vi "Topo & GridSpectr_DriftCorrection_zSpec_v13.vi"(6 "Internal use":string, 7 "Grid param":T1 {"height (m)" format="%#_6p"; "width (m)" format="%#_6p"; "center Y (m)" format="%#_6p"; "center X (m)" format="%#_6p"}, 8 "Error in (no error)":errorcluster, 9 "Points Y/Index Y":i32, 10 "Points X/Index X":i32, 11 "Method":enum16{"init", "run", "end"}(ring)=enum."end") -> (0 "Error out":errorcluster)   [LabVIEW 2014]
doc: "Example of a measurement VI to be used in the \"Experiments on a Grid\" tool as external VI.\n\nThis example measure the topography and spectroscopy data. The spectroscopy measurements are taken on a subgrid. The data are saved to a sxm and a binary file.\n\n- Nanonis Programming Interface -"
uses:
  <userlib>/Nanonis Prog Interface V5/Scan/Grid/GridPatternGet.vi
  <userlib>/Nanonis Prog Interface V5/Scan/Grid/LinePatternGet.vi
  <userlib>/Nanonis Prog Interface V5/Nanonis Prog Interface.lvlib
panel:
  in  "during Spec Bias (V)":sgl=-0.00027 format="%#_5p"
  in  "type":u16(ring)=1 items=["Line", "Grid"]
  in  "readjust setpoint every":i32=4
  in  "Correct Drift":bool=TRUE
  in  "Email when finished":string="cornelius.krull@monash.edu"
  in  "STS z offset":dbl format="%#_6p"
  out "ETA":timestamp=timestamp(3568104746.9132867 s since 1904-01-01)
  out "remaining":dbl format="%<%H:%M:%S>t"
  out "Progress":u8(slide)=100 scale=0.0..100.0 scale format="%#.1g"
  out "total Points":i32=960
  in  "preSTS delay [ms]":u32=500
  in  "ref Bias":dbl=0.02 format="%#_6p"
  in  "Imaging Bias":dbl=0.02 format="%#_6p"
  in  "max applied Drift Correction":i32=20 min=1 max=100 step=1 format="%.0p"
  in  "Correlate":u16(ring) items=["first Frame", "successive Frames"]
  out "Topo Images taken":i32=47
  in  "Increment":i32=20
  in  "Threshold":i32=2 min=1 step=1
  in  "tip Speed (m/s)":sgl=2e-09 format="%.2p"
  out "X drift":i32=2
  out "Y drift":i32=-2
  out "Last Drift detected":i32=1
  in  "MaxImagesBack":i32=2
  in  "Channel index (0-23)":u8(ring) items=["Current"=0, "Z (m)"=14]
  in  "File name":string="symmetric_node"
  in  "ref Current":dbl=5e-12 format="%#_6p"
  in  "Imaging Current":dbl=5e-12 format="%#_6p"
  in  "zdrift \nDuration (s)":dbl
  in  "Correct z drift":bool
  out "Status":string="finishing"
  in  "Drift correction Pixels":i32=256 caption="Topo Pixels"
  out "Y Offset":dbl=3.096245239364581e-10 format="%#_6p"
  out "X Offset":dbl=3.3116363991336772e-09 format="%#_6p"
  out "Points taken":dbl=960.0
  in  "Drift Correction every":i32=20
  in  "Y subgrid spacing":u16=1
  in  "X subgrid spacing":u16=1
  # "z Spectroscopy"
  # "GRID points"
  # "Increase this if no Drift was detected for \na certain number of images"
  # "%"
  # "time (HH:MM:SS)"
  # "images back"
  # "% of image size"
  # "RUN smart tilt before starting the GRID\nImg Angle = 0\nmove tip to reference point for tip height"
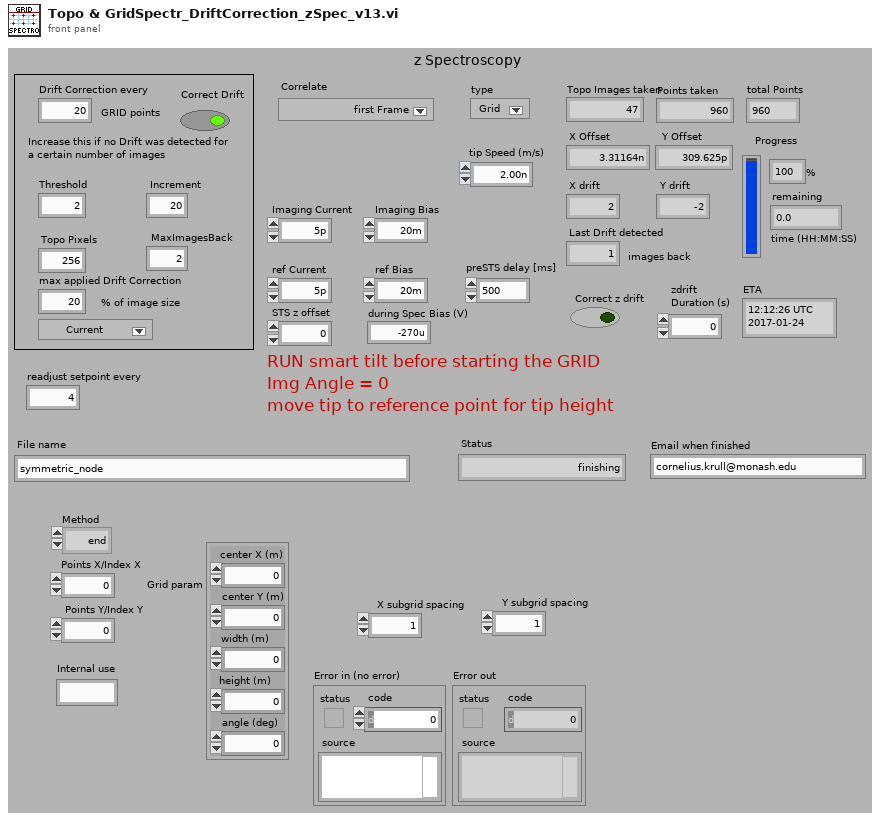
[diagram p1: front panel]
types:
  T1 = cluster{"center X (m)":sgl, "center Y (m)":sgl, "width (m)":sgl, "height (m)":sgl, "angle (deg)":sgl}
  T2 = cluster{"Z averaging time (s)":sgl, "Z offset (m)":sgl, "Initial settling time (s)":sgl}
  T3 = cluster{"Drift correction Pixels":i32, "Imaging Current":dbl, "STS Current":dbl, "MaxImagesBack":i32, "tip Speed (m/s)":sgl, "Threshold":i32, "Increment":i32, "Correlate":u16, "max applied Drift Correction":i32, "Imaging Bias":dbl, "Move Current":dbl, "Move Bias":dbl, "STS Bias":dbl, "preSTS delay [ms]":u32, "STS z offset":dbl, "Correct Drift":bool, "Lockin ON/OFF":bool}
  T4 = cluster{"center X":sgl, "center Y":sgl, "angle":sgl, "width":sgl, "height":sgl, "# pixels":i32, "# lines":i32}
  T5 = cluster{"Name":string, "Calibration":sgl, "Offset":sgl, "Channel index":i32}[]
  T6 = cluster{"up/down":bool, "time/line":sgl, "start time":timestamp, "end time":timestamp}
  T7 = cluster{"Z averaging time (s)":sgl, "Initial settling time (s)":sgl}
  T8 = cluster{"Max. slew rate (m/s)":sgl, "Settling time (s)":sgl, "Integration time (s)":sgl}
  T9 = cluster{"End settling time (s)":sgl, "Z control time (s)":sgl}
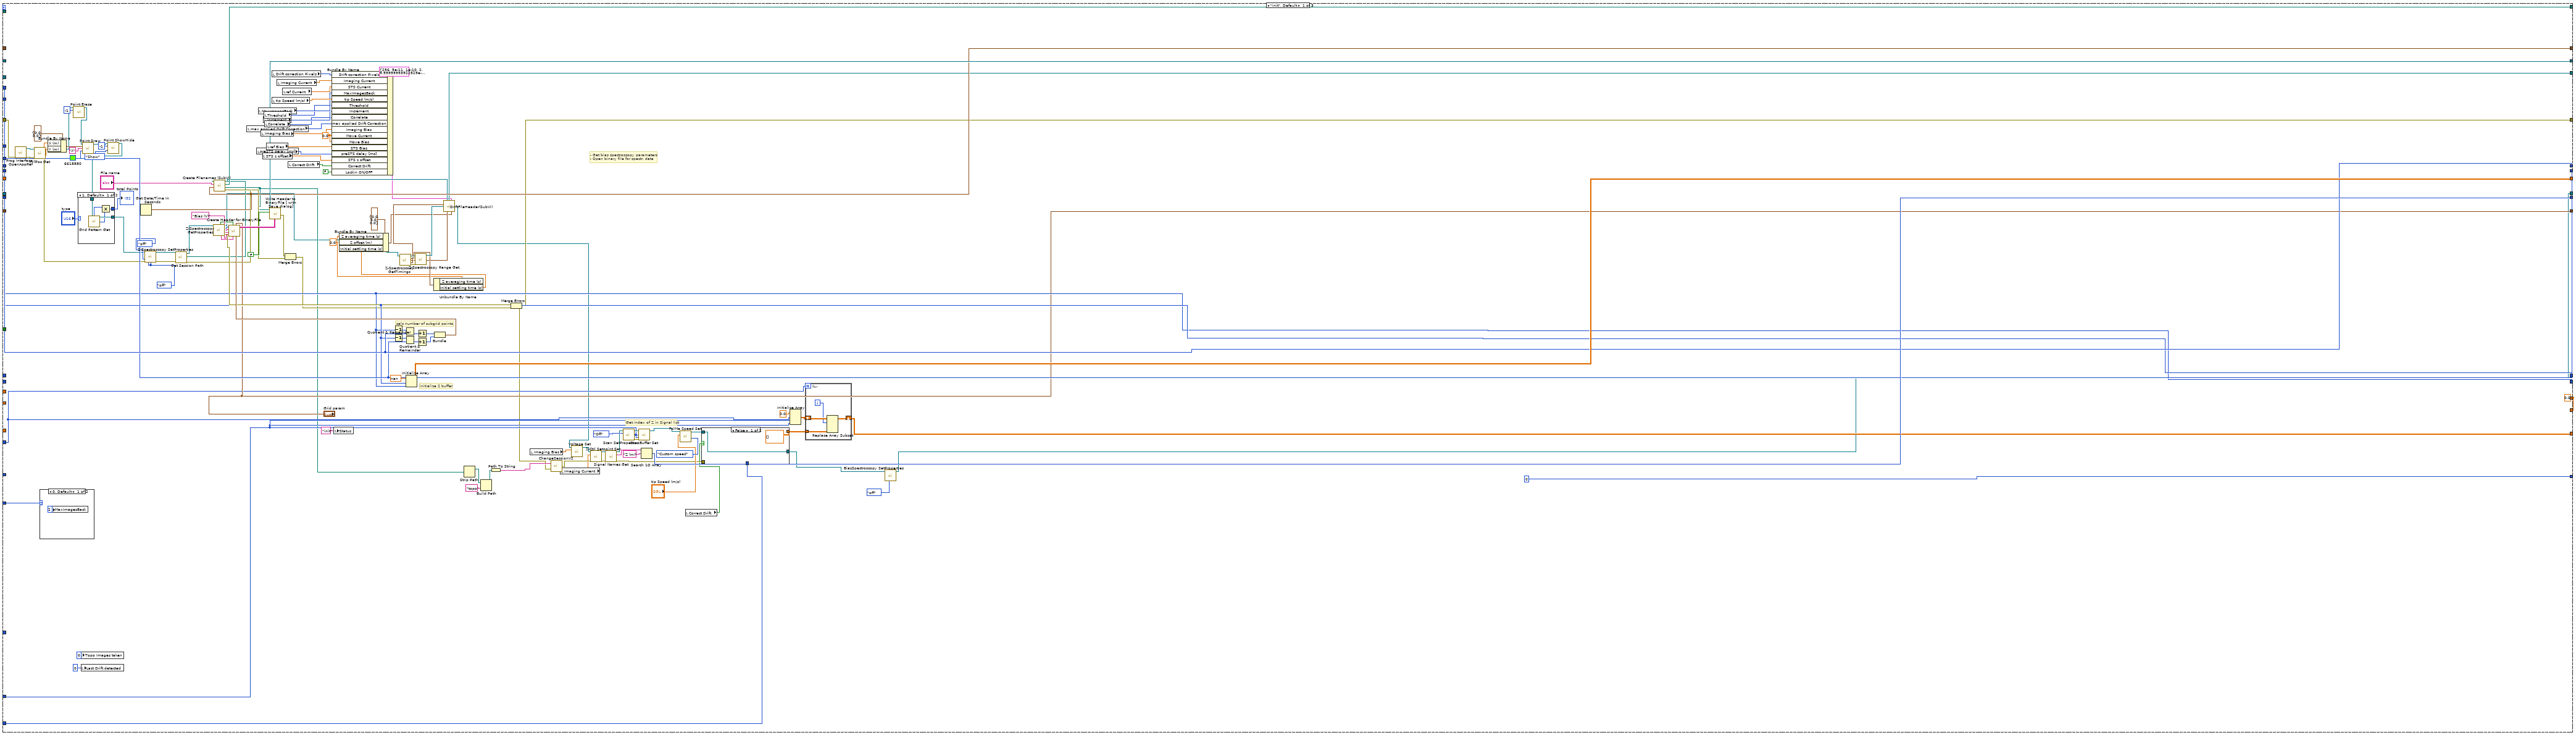
[diagram p2: hidden frame]
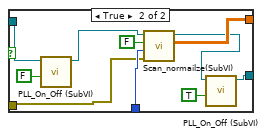
[diagram p3: hidden frame]
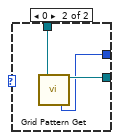
[diagram p4: hidden frame]
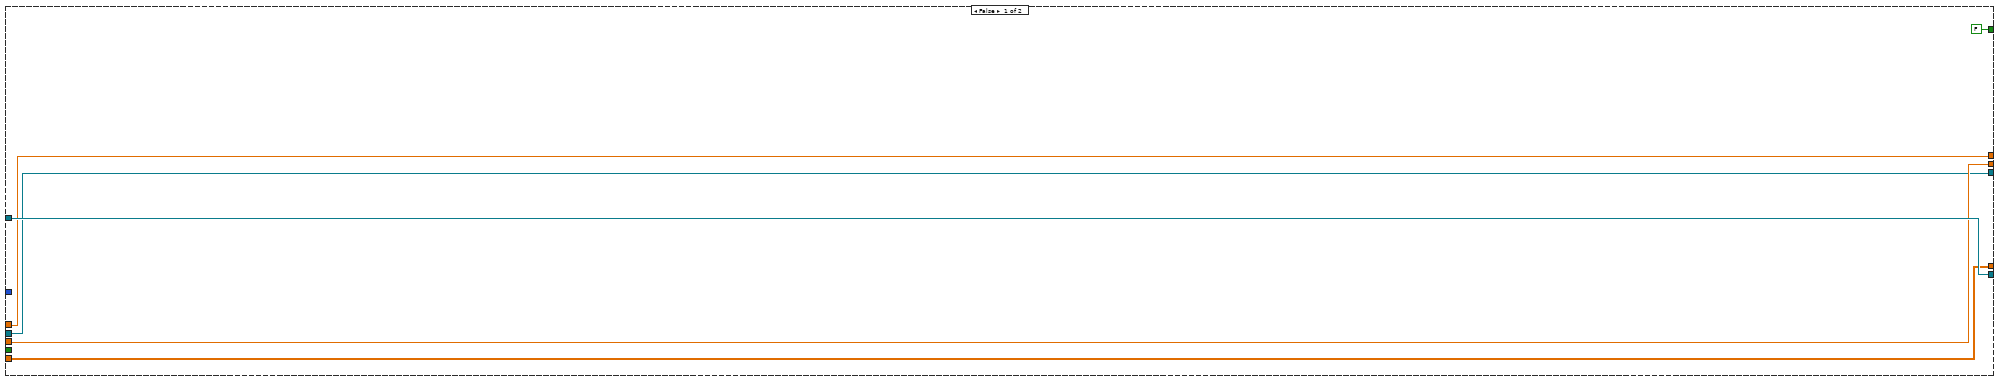
[diagram p9: hidden frame]
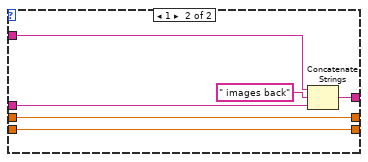
[diagram p10: hidden frame]
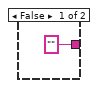
[diagram p12: hidden frame]
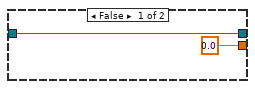
[diagram p13: hidden frame]
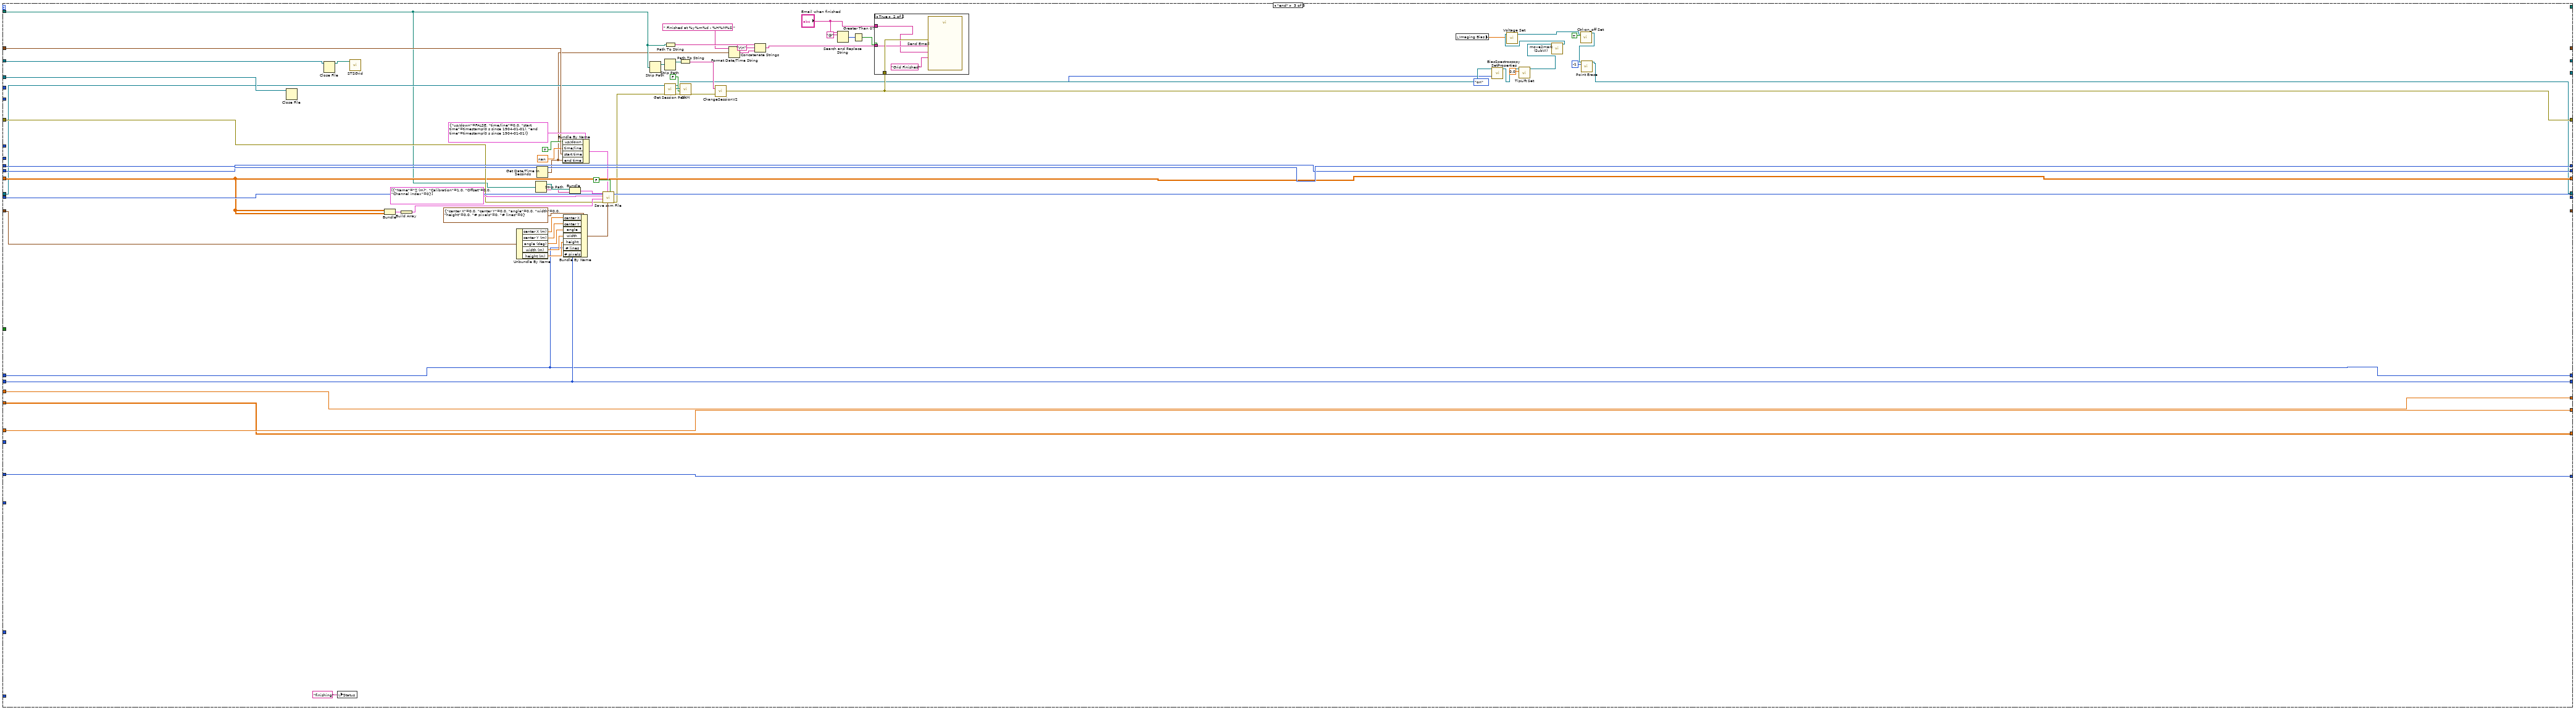
[diagram p15: hidden frame]
diagram:
  # "This string control is required so this VI's connector is compatible with the Nanonis module : \"Experiment on a grid\"."
  # "IMPORTANT : The connector of your own VI must EXACTLY match the connector of this example VI.\n\nThis example VI will do the following:\n- init: Open/Create a sxm (scan data file). Store file path in shift register. Initialize buffer for the topography data. Open binary file and create header.\n- run: Get Z position and write it to topography buffer (from last row to first row of buffer, to make it compatible to Save sxm File function which assumes data starting on the top left corner of image). If grid indices x,y are multiples of the subgrid spacings, start a bias spectroscopy experiment. Write the spectroscopy data to the binary file.\n- end: Write data from topography buffer to file, along with grid dimensions and other known parameters. Close files."
  n1 = while {
    shift-right: [w21] -> _
    shift-left: _ -> [w44]
    shift-right: [w39] -> _
    shift-left: _ -> [w38]
    shift-right: [w36] -> _
    shift-left: _ -> [w37]
    shift-right: [w35] -> _
    shift-left: _ -> [w34]
    shift-right: [w28] -> _
    shift-left: _ -> [w30]
    shift-right: [w29] -> _
    shift-left: _ -> [w31]
    shift-right: [w27] -> _
    shift-left: _ -> [w26]
    shift-right: [w25] -> _
    shift-left: _ -> [w24]
    shift-right: [w23] -> _
    shift-left: _ -> [w22]
    shift-right: [w20] -> _
    shift-left: _ -> [w19]
    shift-right: [w18] -> _
    shift-left: _ -> [w17]
    shift-right: [w16] -> _
    shift-left: _ -> [w9]
    shift-right: [w15] -> _
    shift-left: _ -> [w8]
    shift-right: [w14] -> _
    shift-left: _ -> [w11]
    shift-right: [w13] -> _
    shift-left: _ -> [w10]
    shift-right: [w6] -> _
    shift-left: _ -> [w5]
    stop <- TRUE stop-if-true
    # "> Drift file ref >"
    # "> number of  points  >"
    # "> Ref Frame  >"
    # "> Grid param >"
    # "> start time >"
    # ">Application reference >"
    # "> Y Subgrid spacing >"
    # "> X Subgrid spacing >"
    # "> Z signal index >"
    # "> Binary file ref >"
    # "> Z buffer >"
    # "> sxm file path >"
    n2 = case shown="\"run\"" "Method" {
      tunnel: [w139 w273 _] -> w21
      tunnel: w44 -> [_ w273 w449]
      tunnel: "Error in (no error)" -> [w141 w259 w480]
      tunnel: [w120 w272 w450] -> w42
      tunnel: "Points X/Index X" -> [w153 w267 _]
      tunnel: "Points Y/Index Y" -> [w154 w252 _]
      tunnel: [w177 w270 w469] -> w39
      tunnel: w38 -> [_ w271 w469]
      tunnel: w37 -> [_ w269 w462]
      tunnel: [w169 w268 _] -> w36
      tunnel: [w167 w257 w494] -> w35
      tunnel: w34 -> [_ w257 w494]
      tunnel: "X subgrid spacing" -> [w166 _ _]
      tunnel: "Y subgrid spacing" -> [w165 _ _]
      tunnel: w31 -> [_ w261 w493]
      tunnel: w30 -> [_ w260 w492]
      tunnel: [w166 w261 w493] -> w29
      tunnel: [w165 w260 w492] -> w28
      tunnel: [w105 w245 w433] -> w27
      tunnel: w26 -> [_ w229 w455]
      tunnel: ["Grid param" w255 _] -> w25
      tunnel: w24 -> [_ w255 w479]
      tunnel: [w138 w220 _] -> w23
      tunnel: w22 -> [_ w220 w487]
      tunnel: [w154 w253 w470] -> w20
      tunnel: w19 -> [_ w253 w470]
      tunnel: [w153 w254 w471] -> w18
      tunnel: w17 -> [_ w254 w471]
      tunnel: [w150 w235 w468] -> w16
      tunnel: [w150 w240 w466] -> w15
      tunnel: [w134 w234 w463] -> w14
      tunnel: [0 w218 w467] -> w13
      tunnel: w10 -> [_ w204 w467]
      tunnel: "Drift Correction every" -> [_ w248 _]
      tunnel: w11 -> [_ w239 w463]
      tunnel: w9 -> [_ w246 w468]
      tunnel: w8 -> [_ w232 w466]
      tunnel: "Drift correction Pixels" -> [w133 _ _]
      tunnel: [w101 w237 _] -> w6
      tunnel: w5 -> [_ w238 w464]
      tunnel: "Correct z drift" -> [_ w236 _]
      tunnel: "Channel index (0-23)" -> [w83 w233 _]
      tunnel: "MaxImagesBack" -> [w132 _ _]
      tunnel: "Correlate" -> [w113 _ _]
      frame "init", Default {
        w48 = 0.0 ("Move Current")
        w103 = enum16{"no change", "on", "off"}."off" ("Save dialog")
        w150 = 0.0
        # "- Get bias spectroscopy parameters\n- Open binary file for spectr. data"
        # "initialize Z buffer"
        # "calc number of subgrid points"
        # "Get index of Z in Signal list"
        n3 = call <userlib>:"Prog Interface - OpenAppRef.vi"("Error in (no error)"=w141) -> ("Error out"=w78:errorcluster, "Application reference"=w80:refnum<vi>)  [unwired: 5 in]
        n4 = call <userlib>:"XY-Pos Get.vi"("error in (no error)"=w78, "Application ref in"=w80) -> ("error out"=w79:errorcluster, "Y (m)"=w72:sgl, "X (m)"=w73:sgl, "Application ref out"=w54:refnum<vi>)  [unwired: 5 in]
        n5 = case shown="0, Default" w113 {
          frame 0, Default {
            n6 = local write "MaxImagesBack"(2 ("StepsBack")) -> ()
          }
          frame 1 {
          }
        }
        n7 = Bundle By Name(cluster=cluster{"X (m)":sgl, "Y (m)":sgl} {"X (m)"=0.0, "Y (m)"=0.0} ("Point Coordinates"), "X (m)"=w73, "Y (m)"=w72) -> (w74:cluster{"X (m)":sgl, "Y (m)":sgl})
        n8 = call <userlib>:"Point Erase.vi"("Application ref in"=w54, "Point index (-1=All points)"=-1) -> ("Application ref out"=w53:refnum<vi>)  [unwired: 12 in, 1 out]
        n9 = local write "Topo Images taken"(0 ("Images taken")) -> ()
        n10 = local write "Last Drift detected"(0 ("Last Drift detected")) -> ()
        n11 = call <userlib>:"Point Draw.vi"("Application ref in"=w53, "Point Coordinates"=w74, "Text"="X", "Color"=u32 6618880) -> ("Application ref out"=w58:refnum<vi>)  [unwired: 10 in, 1 out]
        n12 = call <userlib>:"Point ShowHide.vi"("Application ref in"=w58, "Point index (-1=All points)"=-1, "Show/Hide"=enum16{"Show", "Hide"}."Show") -> ("Application ref out"=w57:refnum<vi>)  [unwired: 11 in, 1 out]
        n13 = case shown="1, Default" "type" {
          tunnel: [w194 w197] -> w107
          tunnel: [w191 w195] -> w106
          tunnel: w57 -> [w190 w196]
          frame 1, Default {
            n14 = call-poly <userlib>:"Grid Pattern Get.vi"("Application ref in"=w190) -> ("Points Y"=w192:i32, "Points X"=w193:i32, "Application ref out"=w194:refnum<vi>)  [unwired: 10 in, 6 out]
            n15 = Multiply(x=w192, y=w193) -> (x*y=w191:i32)
          }
          frame 0 {
            n16 = call-poly <userlib>:"Grid Pattern Get.vi"("Application ref in"=w196) -> ("Points"=w195:i32, "Application ref out"=w197:refnum<vi>)  [unwired: 12 in, 5 out]
          }
        }
        "total Points" <- w106
        n17 = Get Date/Time In Seconds() -> (seconds since 1Jan1904=w138:timestamp)
        n18 = call <userlib>:"Z-Spectroscopy SetProperties.vi"("Application ref in"=w107, "Autosave"=enum16{"no change", "on", "off"}."off" ("Autosave (no change)"), "error in (no error)"=w79, "Save dialog"=w103, "Save all sweeps (no change)"=w103) -> ("Application ref out"=w116:refnum<vi>, "error out"=w115:errorcluster)  [unwired: 9 in]
        n19 = call <userlib>:"Get Session Path.vi"("error in (no error)"=w115, "Application ref in"=w116) -> ("error out"=w140:errorcluster, "Session path"=w126:path, "Application ref out"=w117:refnum<vi>)  [unwired: 7 in]
        n20 = call <userlib>:"Z-Spectroscopy GetProperties.vi"("Application ref in"=w117) -> ("Backward sweep"=w173:bool, "Application ref out"=w69:refnum<vi>, "Number of points"=w156:i32, "Channels"=w155:string[], "Parameters"=w171:string[], "Fixed parameters"=w158:string[], "error out"=w170:errorcluster)  [unwired: 7 in, 1 out]
        n21 = call "Create Filenames (SubVI).vi"("error in (no error)"=w140, "seconds since 1Jan1904"=w138, "File name"="File name", "Session path"=w126) -> ("error out"=w129:errorcluster, "binFilePath"=w122:path, "topoFilePath"=w139:path, "Drift File out"=w102:refnum<file>)  [unwired: 4 in]
        n22 = local read "max applied Drift Correction"() -> (w89:i32)
        n23 = local read "preSTS delay [ms]"() -> (w86:u32)
        n24 = local read "MaxImagesBack"() -> (w93:i32)
        n25 = local read "Imaging Bias"() -> (w88:dbl)
        n26 = local read "STS z offset"() -> (w85:dbl)
        n27 = local read "Increment"() -> (w91:i32)
        n28 = local read "Threshold"() -> (w92:i32)
        n29 = local read "Correlate"() -> (w90:u16)
        n30 = local read "ref Bias"() -> (w87:dbl)
        n31 = local read "Drift correction Pixels"() -> (w97:i32)
        n32 = local read "tip Speed (m/s)"() -> (w94:sgl)
        n33 = local read "Imaging Current"() -> (w96:dbl)
        n34 = local read "ref Current"() -> (w95:dbl)
        n35 = local read "Correct Drift"() -> (w84:bool)
        n36 = Bundle By Name(cluster=T3 {"Drift correction Pixels"=256, "Imaging Current"=5e-11, "STS Current"=1e-10, "MaxImagesBack"=2, "tip Speed (m/s)"=1e-08, "Threshold"=2, "Increment"=64, "Correlate"=0, "max applied Drift Correction"=20, "Imaging Bias"=-0.02, "Move Current"=1.5e-11, "Move Bias"=-0.02, "STS Bias"=0.1, "preSTS delay [ms]"=1000, "STS z offset"=-1.7e-10, "Correct Drift"=TRUE, "Lockin ON/OFF"=TRUE} ("Drift Correction"), "Drift correction Pixels"=w97, "Imaging Current"=w96, "STS Current"=w95, "MaxImagesBack"=w93, "tip Speed (m/s)"=w94, "Threshold"=w92, "Increment"=w91, "Correlate"=w90, "max applied Drift Correction"=w89, "Imaging Bias"=w88, "Move Current"=w48, "Move Bias"=w48, "STS Bias"=w87, "preSTS delay [ms]"=w86, "STS z offset"=w85, "Correct Drift"=w84, "Lockin ON/OFF"=FALSE) -> (w99:T3)
        n37 = local write "Status"("init" ("Status")) -> ()
        n38 = Decrement(x=w153) -> (x-1=w164:i32)
        n39 = Decrement(x=w154) -> (x-1=w163:i32)
        n40 = call <userlib>:"Z-Spectroscopy GetTimings.vi"("Application ref in"=w69) -> ("Application ref out"=w70:refnum<vi>, "Initialization"=w65:T7, "Sweep Timing"=w66:T8, "End of Sweep"=w67:T9, "Error out"=w71:errorcluster)  [unwired: 10 in]
        n41 = Quotient & Remainder(x=w164, y=w166) -> (floor(x/y)=w162:i32)  [unwired: 1 out]
        n42 = Quotient & Remainder(x=w163, y=w165) -> (floor(x/y)=w161:i32)  [unwired: 1 out]
        n43 = Initialize Array(sgl nan ("element"), w154, w153) -> (w177:sgl[][])
        n44 = call <userlib>:"Z-Spectroscopy Range Get.vi"("error in (no error)"=w71, "Application ref in"=w70) -> ("Application ref out"=w68:refnum<vi>)  [unwired: 5 in, 3 out]
        n45 = Increment(x=w162) -> (x+1=w160:i32)
        n46 = Increment(x=w161) -> (x+1=w159:i32)
        n47 = Unbundle By Name(w65) -> ("Z averaging time (s)"=w62:sgl, "Initial settling time (s)"=w61:sgl)
        n48 = Bundle By Name(cluster=T2 {"Z averaging time (s)"=0.0, "Z offset (m)"=0.0, "Initial settling time (s)"=0.0} ("Initialization"), "Z averaging time (s)"=w62, "Z offset (m)"=sgl 0.0, "Initial settling time (s)"=w61) -> (w63:T2)
        n49 = Bundle(w160, w159) -> (w172:cluster{i32, i32})  [unwired: 1 in]
        n50 = call <userlib>:"Create Header for BinaryFile.vi"("Grid points"=w172, "Grid param"="Grid param", "Fixed parameters"=w158, "Backward sweep"=w173, "Sweep signal"="Bias (V)" ("Sweep Signal"), "Parameters"=w171, "Channels"=w155, "Points per sweep"=w156) -> ("Header (fixed attributes)"=w175:string[][])  [unwired: 3 in]
        n51 = call <userlib>:"Write Header to BinaryFile [ with Save dialog].vi"("Fixed Attributes"=w175, "Show Dialog? (T)"=FALSE, "Filename"=w122) -> ("Error out"=w130:errorcluster, "File ref"=w169:refnum<file>)  [unwired: 5 in, 2 out]
        n52 = Merge Errors(w130, w129) -> (w131:errorcluster)
        n53 = call "DriftFileHeader(SubVI).vi"("Byte Stream File in"=w102, "Drift Correction"=w99, "End of Sweep"=w67, "Application ref in"=w68, "Sweep Timing"=w66, "Initialization"=w63) -> ("Byte Stream File out"=w101:refnum<file>, "Application ref out"=w100:refnum<vi>)  [unwired: 8 in]
        n54 = Strip Path(path=w122) -> (stripped path=w125:path)  [unwired: 1 out]
        n55 = Build Path(base path=w125, name or relative path="topo") -> (appended path=w123:path)
        n56 = Path To String(path=w123) -> (string=w121:string)
        n57 = Merge Errors(w170, w131) -> (w120:errorcluster)
        n58 = local read "Imaging Bias"() -> (w109:dbl)
        n59 = call "ChangeSessionV2.vi"("error in (no error)"=w120, "Session"=w121) -> ("error out"=w119:errorcluster)
        n60 = local read "Imaging Current"() -> (w108:dbl)
        n61 = call <userlib>:"Voltage Set.vi"("Bias (V)"=w109, "Application ref in"=w100) -> ("Application ref out"=w110:refnum<vi>)  [unwired: 8 in, 1 out]
        n62 = call <userlib>:"Z-Ctrl Setpoint Set.vi"("error in (no error)"=w119, "Z Controller setpoint"=w108, "Application ref in"=w110) -> ("error out"=w142:errorcluster, "Application ref out"=w143:refnum<vi>)  [unwired: 7 in]
        n63 = call <userlib>:"Signal Names Get.vi"("error in (no error)"=w142, "Application ref in"=w143) -> ("error out"=w82:errorcluster, "Signals Names"=w157:string[], "Application ref out"=w146:refnum<vi>)  [unwired: 5 in]
        n64 = call <userlib>:"Scan SetProperties.vi"("Application ref in"=w146, "Continuous scan"=enum16{"No change", "On", "Off"}."Off") -> ("Application ref out"=w148:refnum<vi>, "Error out"=w147:errorcluster)  [unwired: 12 in]
        n65 = call <userlib>:"ScanBuffer Set.vi"("Application ref in"=w148, "Pixels"=w133, "Lines"=w133, "error in (no error)"=w147) -> ("Application ref out"=w111:refnum<vi>)  [unwired: 10 in, 1 out]
        n66 = Search 1D Array(1D array=w157, element="Z (m)") -> (index of element=w167:i32)  [unwired: 1 in]
        n67 = call <userlib>:"FolMe Speed Set.vi"("Speed Setting (Custom)"=enum32{"Scan speed", "Custom speed"}."Custom speed", "Speed (m/s)"="tip Speed (m/s)", "Application ref in"=w111) -> ("Application ref out"=w51:refnum<vi>)  [unwired: 5 in, 1 out]
        n68 = local read "Correct Drift"() -> (w49:bool)
        n69 = case shown="False" w49 {
          tunnel: w83 -> [_ w189]
          tunnel: w82 -> [_ w188]
          tunnel: [dbl[][] [] ("Array") w187] -> w81
          tunnel: w51 -> [w179 w185]
          tunnel: [w179 w180] -> w47
          frame False {
          }
          frame True {
            n70 = call "PLL_On_Off (SubVI).vi"("Output ON/OFF (F=OFF)"=FALSE, "Application in"=w185) -> ("Application out"=w184:refnum<vi>)  [unwired: 8 in, 1 out]
            n71 = call "Scan_normailze(SubVI).vi"("error in (no error)"=w188, "Channel index (0-23)"=w189, "Normalization"=FALSE ("Boolean"), "Application in"=w184) -> ("Array"=w187:dbl[][], "Application out"=w181:refnum<vi>)  [unwired: 5 in, 1 out]
            n72 = call "PLL_On_Off (SubVI).vi"("Output ON/OFF (F=OFF)"=TRUE, "Application in"=w181) -> ("Application out"=w180:refnum<vi>)  [unwired: 8 in, 1 out]
          }
        }
        n73 = Initialize Array(0.0 ("element"), w132, w133, w133) -> (w135:dbl[][][])
        n74 = for {
          N: w132 -> [_]
          tunnel: w81 -> [w201]
          shift-right: [w200] -> w134
          shift-left: w135 -> [w202]
          i -> [w199]
          n75 = Replace Array Subset(array=w202, new element=w201, index (dim 0)=w199) -> (w200:dbl[][][])  [unwired: 2 in]
        }
        n76 = call <userlib>:"BiasSpectroscopy SetProperties.vi"("Application ref in"=w47, "Z-Controller hold (no change)"=enum16{"no change", "on", "off"}."off") -> ("Application ref out"=w105:refnum<vi>)  [unwired: 12 in, 1 out]
      }
      frame "run" {
        # "shift tip position"
        # "Get Z position"
        # "- get Z position for topography and store it to Z buffer\n- if x,y indices are a multiple of the spacings, take spectroscopy curve and write data to binary file\ndo drift correction if number of STS position was reached"
        n77 = local read "Correct Drift"() -> (w212:bool)
        n78 = Quotient & Remainder(x=w204, y=w248) -> (x-y*floor(x/y)=w249:i32)  [unwired: 1 out]
        n79 = Not Equal To 0?(x=w204) -> (x != 0?=w230:bool)
        n80 = Equal To 0?(x=w249) -> (x = 0?=w247:bool)
        n81 = call <userlib>:"XY-Pos Get.vi"("Wait for newest data (F=False)"=TRUE, "Application ref in"=w229) -> ("Y (m)"=w225:sgl, "X (m)"=w226:sgl, "Application ref out"=w228:refnum<vi>)  [unwired: 5 in, 1 out]
        n82 = Compound Arithmetic op=AND(w230, w247, w212) -> (w231:bool)
        n83 = case shown="True" w231 {
          tunnel: w228 -> [w314 w325]
          tunnel: [w314 w370] -> w209
          tunnel: w239 -> [w311 w366]
          tunnel: [w313 w368] -> w235
          tunnel: [w312 w367] -> w240
          tunnel: w246 -> [w313 w349]
          tunnel: w232 -> [w312 w347]
          tunnel: [w311 w362] -> w234
          tunnel: w238 -> [w310 w373]
          tunnel: [w310 w372] -> w237
          tunnel: w236 -> [_ w369]
          tunnel: w233 -> [_ w353]
          tunnel: [FALSE TRUE] -> w206
          frame False {
          }
          frame True {
            # "Drift correction \ncompare to the reference image with the previous image \ndx and dy will be applied to the grid coord, \nand the imaging frame will be shifted"
            n84 = Greater Or Equal To 0?(x=w353) -> (x >= 0?=w352:bool)
            n85 = call "move2mark (SubVI).vi"("Application in"=w325) -> ("Application out"=w324:refnum<vi>)  [unwired: 10 in]
            n86 = local write "Status"("Drift Correction" ("Status")) -> ()
            n87 = case shown="True" w352 {
              frame False {
              }
              frame True {
                n88 = local read "Topo Images taken"() -> (w388:i32)
                n89 = Increment(x=w388) -> (x+1=w387:i32)
                n90 = local write "Topo Images taken"(w387) -> ()
              }
            }
            n91 = local read "Imaging Bias"() -> (w332:dbl)
            n92 = call <userlib>:"Voltage Set.vi"("Bias (V)"=w332, "Application ref in"=w324) -> ("Application ref out"=w333:refnum<vi>)  [unwired: 8 in, 1 out]
            n93 = local read "Imaging Current"() -> (w331:dbl)
            n94 = call <userlib>:"Z-Ctrl Setpoint Set.vi"("Z Controller setpoint"=w331, "Application ref in"=w333) -> ("Application ref out"=w323:refnum<vi>)  [unwired: 8 in, 1 out]
            n95 = call <userlib>:"Ctrl-on_off Set.vi"("Z Controller ON/OFF"=TRUE, "Application ref in"=w323) -> ("Application ref out"=w321:refnum<vi>)  [unwired: 8 in, 1 out]
            n96 = call "PLL_On_Off (SubVI).vi"("Output ON/OFF (F=OFF)"=FALSE, "Application in"=w321) -> ("Application out"=w320:refnum<vi>)  [unwired: 8 in, 1 out]
            n97 = call "Scan_normailze(SubVI).vi"("Channel index (0-23)"=w353, "Normalization"=FALSE ("Boolean"), "Application in"=w320) -> ("Array"=w363:dbl[][], "Application out"=w318:refnum<vi>)  [unwired: 6 in, 1 out]
            n98 = Divide(x="max applied Drift Correction", y=100) -> (x/y=w340:dbl)
            n99 = local read "Drift correction Pixels"() -> (w341:i32)
            n100 = local read "Last Drift detected"() -> (w344:i32)
            n101 = local read "Correlate"() -> (w350:u16)
            n102 = call "PLL_On_Off (SubVI).vi"("Output ON/OFF (F=OFF)"=TRUE, "Application in"=w318) -> ("Application out"=w315:refnum<vi>)  [unwired: 8 in, 1 out]
            n103 = Multiply(x=w340, y=w341) -> (x*y=w342:dbl)
            n104 = call "CorrelImages (SubVI)v2.vi"("last drift detected"=w344, "Correlate"=w350, "Ref Array"=w366, "New Image"=w363) -> ("Y drift"=w338:i32, "X drift"=w335:i32, "Ref Array out"=w362:dbl[][][], "Queue Steps"=w351:i32)  [unwired: 4 in]
            "X drift" <- w335
            "Y drift" <- w338
            "Last Drift detected" <- w351
            n105 = local read "Topo Images taken"() -> (w355:i32)
            n106 = To Long Integer(number=w342) -> (32bit integer=w334:i32)
            n107 = Greater Or Equal?(x=w351, y="Threshold") -> (x >= y?=w357:bool)
            n108 = Greater?(x=w355, y="Threshold") -> (0:w354:bool)
            n109 = call "AbsLimit (SubVI).vi"("in"=w335, "Abslimt"=w334) -> ("Numeric out"=w337:i32)  [unwired: 9 in]
            n110 = call "AbsLimit (SubVI).vi"("in"=w338, "Abslimt"=w334) -> ("Numeric out"=w336:i32)  [unwired: 9 in]
            n111 = And(x=w357, y=w354) -> (x .and. y?=w356:bool)
            n112 = case shown="True" w356 {
              tunnel: ["" w392] -> w358
              frame False {
              }
              frame True {
                n113 = local read "Drift Correction every"() -> (w391:i32)
                n114 = local write "Last Drift detected"(0 ("Last Drift detected")) -> ()
                n115 = Add(x=w391, y="Increment") -> (x+y=w395:i32)
                n116 = local write "Drift Correction every"(w395) -> ()
                n117 = Number To Decimal String(number=w395) -> (decimal integer string=w394:string)  [unwired: 1 in]
                n118 = Concatenate Strings(" Increased DC to every " ("string"), w394) -> (w392:string)
              }
            }
            n119 = local read "Drift correction Pixels"() -> (w360:i32)
            n120 = Number To Decimal String(number=w351) -> (decimal integer string=w365:string)  [unwired: 1 in]
            n121 = case shown="0, Default" w350 {
              tunnel: w365 -> [w375 w386]
              tunnel: [w380 w385] -> w364
              tunnel: w358 -> [w378 w383]
              tunnel: w349 -> [w376 w382]
              tunnel: [w376 w382] -> w348
              tunnel: w347 -> [w377 w381]
              tunnel: [w377 w381] -> w346
              frame 0, Default {
                n122 = Concatenate Strings(w375, "images back , Correlating first frame " ("string"), w378) -> (w380:string)
              }
              frame 1 {
                n123 = Concatenate Strings(w386, " images back" ("string"), w383) -> (w385:string)
              }
            }
            n124 = call "drift_pixel2m (SubVI).vi"("Application in"=w315, "X drift"=w337, "Y drift"=w336, "Drift correction Pixels"=w360) -> ("Application out"=w359:refnum<vi>, "x drift"=w329:sgl, "y drift"=w328:sgl)  [unwired: 2 in, 1 out]
            n125 = call "ShiftFrame (SubVI).vi"("Y shift"=w328, "X shift"=w329, "Application in"=w359) -> ("Application out"=w361:refnum<vi>)  [unwired: 8 in]
            n126 = call "MoveGrid.vi"("y"=w328, "x"=w329, "Application ref in"=w361) -> ("Application ref out"=w327:refnum<vi>)  [unwired: 7 in, 1 out]
            n127 = call "shift marks (SubVI).vi"("y"=w328, "x"=w329, "Application in"=w327) -> ("Application out"=w326:refnum<vi>)  [unwired: 7 in, 1 out]
            n128 = case shown="True" w369 {
              tunnel: [0.0 ("z drift") w402] -> w371
              tunnel: w326 -> [w397 w401]
              tunnel: [w397 w400] -> w370
              frame False {
              }
              frame True {
                n129 = call "Zdrift_subVi.vi"("Duration"="zdrift \nDuration (s)", "Application in"=w401) -> ("z drift"=w402:dbl, "Application out"=w400:refnum<vi>)  [unwired: 7 in, 1 out]
              }
            }
            n130 = Add(x=w348, y=w329) -> (x+y=w368:dbl)
            n131 = Add(x=w328, y=w346) -> (x+y=w367:dbl)
            n132 = local write "X Offset"(w368) -> ()
            n133 = local write "Y Offset"(w367) -> ()
            n134 = call "Drift Data to file (SubVI).vi"("z drift"=w371, "Comment"=w364, "y Drift"=w367, "X drift"=w368, "Byte Stream File in"=w373) -> ("Byte Stream File out"=w372:refnum<file>)  [unwired: 6 in]
          }
        }
        n135 = Quotient & Remainder(x=w204, y="readjust setpoint every") -> (x-y*floor(x/y)=w205:i32)  [unwired: 1 out]
        n136 = Equal To 0?(x=w204) -> (x = 0?=w203:bool)
        n137 = Equal To 0?(x=w205) -> (x = 0?=w208:bool)
        n138 = Compound Arithmetic op=OR(w203, w206, w208) -> (w207:bool)
        n139 = case shown="True" w207 {
          tunnel: [w274 w282] -> w210
          tunnel: w209 -> [w274 w287]
          frame False {
          }
          frame True {
            n140 = call "move2mark (SubVI).vi"("Application in"=w287) -> ("Application out"=w286:refnum<vi>)  [unwired: 10 in]
            n141 = local write "Status"("adjust setpoint" ("Status")) -> ()
            n142 = local read "ref Bias"() -> (w285:dbl)
            n143 = local read "ref Current"() -> (w281:dbl)
            n144 = call <userlib>:"Voltage Set.vi"("Bias (V)"=w285, "Application ref in"=w286) -> ("Application ref out"=w283:refnum<vi>)  [unwired: 8 in, 1 out]
            n145 = flat-sequence {
              tunnel: w283 -> [w292]
              tunnel: [w289] -> w280
              tunnel: w281 -> [w291]
              tunnel: w280 -> [w295]
              tunnel: [w295] -> w279
              tunnel: "preSTS delay [ms]" -> [w293]
              tunnel: w279 -> [w300]
              tunnel: [w297] -> w284
              tunnel: [w298] -> w277
              tunnel: w284 -> [w304]
              tunnel: "preSTS delay [ms]" -> [w303]
              tunnel: w277 -> [_]
              tunnel: [w304] -> w275
              tunnel: [w306] -> w282
              tunnel: w275 -> [w307]
              frame #0 {
                n146 = call <userlib>:"Z-Ctrl Setpoint Set.vi"("Z Controller setpoint"=w291, "Application ref in"=w292) -> ("Application ref out"=w290:refnum<vi>)  [unwired: 8 in, 1 out]
                n147 = call <userlib>:"Ctrl-on_off Set.vi"("Z Controller ON/OFF"=TRUE, "Application ref in"=w290) -> ("Application ref out"=w289:refnum<vi>)  [unwired: 8 in, 1 out]
              }
              frame #1 {
                n148 = Greater Than 0?(x=w293) -> (x > 0?=w294:bool)
                n149 = case shown="True" w294 {
                  tunnel: w293 -> [_ w296]
                  frame False {
                  }
                  frame True {
                    n150 = Wait (ms)(milliseconds to wait=w296) -> ()  [unwired: 1 out]
                  }
                }
              }
              frame #2 {
                n151 = local read "STS z offset"() -> (w298:dbl)
                n152 = call <userlib>:"TipLift Set.vi"("TipLift (m)"=w298, "Application ref in"=w300) -> ("Application ref out"=w299:refnum<vi>)  [unwired: 8 in, 1 out]
                n153 = call <userlib>:"Ctrl-on_off Set.vi"("Z Controller ON/OFF"=FALSE, "Application ref in"=w299) -> ("Application ref out"=w297:refnum<vi>)  [unwired: 8 in, 1 out]
              }
              frame #3 {
                n154 = Greater Than 0?(x=w303) -> (x > 0?=w302:bool)
                n155 = case shown="True" w302 {
                  tunnel: w303 -> [_ w305]
                  frame False {
                  }
                  frame True {
                    n156 = Wait (ms)(milliseconds to wait=w305) -> ()  [unwired: 1 out]
                  }
                }
              }
              frame #4 {
                n157 = call <userlib>:"Voltage Set.vi"("Bias (V)"="during Spec Bias (V)", "Application ref in"=w307) -> ("Application ref out"=w306:refnum<vi>)  [unwired: 8 in, 1 out]
              }
            }
          }
        }
        n158 = Quotient & Remainder(x=w267, y=w261) -> (x-y*floor(x/y)=w266:i32)  [unwired: 1 out]
        n159 = Quotient & Remainder(x=w252, y=w260) -> (x-y*floor(x/y)=w265:i32)  [unwired: 1 out]
        n160 = Equal To 0?(x=w266) -> (x = 0?=w264:bool)
        n161 = Equal To 0?(x=w265) -> (x = 0?=w263:bool)
        n162 = And(x=w264, y=w263) -> (x .and. y?=w262:bool)
        n163 = Subtract(x=w253, y=w252) -> (x-y=w251:i32)
        n164 = Decrement(x=w251) -> (x-1=w250:i32)
        n165 = Add(x=w226, y=w235) -> (x+y=w242:dbl)
        n166 = Add(x=w225, y=w240) -> (x+y=w241:dbl)
        n167 = call <userlib>:"XY-Pos Set.vi"("Y (m)"=w241, "X (m)"=w242, "Application ref in"=w210) -> ("Application ref out"=w243:refnum<vi>)  [unwired: 5 in, 1 out]
        n168 = call <userlib>:"Signal Value Get (Animation period).vi"("error in (no error)"=w259, "Signal index (0-47)"=w257, "Application ref in"=w243) -> ("error out"=w258:errorcluster, "Signal value"=w256:sgl, "Application ref out"=w244:refnum<vi>)  [unwired: 5 in]
        n169 = Replace Array Subset(array=w271, new element=w256, index (row)=w250, index (col)=w267) -> (w270:sgl[][])
        n170 = call <userlib>:"Points Get.vi"() -> ()  [unwired: 13 in, 3 out]
        n171 = case shown="True" w262 {
          tunnel: [w405 w412] -> w272
          tunnel: w269 -> [w406 w426]
          tunnel: [w406 w424] -> w268
          tunnel: w258 -> [w405 w423]
          tunnel: w244 -> [w404 w407]
          tunnel: [w404 w408] -> w245
          tunnel: [w403 w410] -> w218
          tunnel: w204 -> [w403 w411]
          frame False {
            # "Point indices aren't multiple of subgrid spacing\n=> no spectroscopy at this point"
          }
          frame True {
            # "remove Bias from data"
            n172 = local write "Status"("zSpec" ("Status")) -> ()
            n173 = call <userlib>:"Z-Spectroscopy Start.vi"("Application ref in"=w407, "Get data (F=False)"=TRUE ("Get Data (F)"), "error in (no error)"=w423) -> ("Application ref out"=w408:refnum<vi>, "Data"=w422:sgl[][], "Parameters"=w421:sgl[], "error out"=w414:errorcluster)  [unwired: 8 in, 1 out]
            n174 = Delete From Array(array=w422, length=1, index (row)=0 ("index")) -> (array with subset deleted=w420:sgl[][])  [unwired: 1 in, 1 out]
            n175 = Write to Binary File(file (use dialog)=w426, data=w421, error in=w414, 5:FALSE ("prepend array or string size? (T)")) -> (refnum out=w425:refnum<file>, error out=w413:errorcluster)  [unwired: 2 in, 1 out]
            n176 = Increment(x=w411) -> (x+1=w410:i32)
            n177 = Write to Binary File(file (use dialog)=w425, data=w420, error in=w413, 5:FALSE ("prepend array or string size? (T)")) -> (refnum out=w424:refnum<file>, error out=w412:errorcluster)  [unwired: 2 in, 1 out]
          }
        }
        n178 = Get Date/Time In Seconds() -> (seconds since 1Jan1904=w215:timestamp)
        n179 = local read "total Points"() -> (w221:i32)
        n180 = Subtract(x=w215, y=w220) -> (x-y=w219:dbl)
        n181 = Divide(x=w218, y=w221) -> (x/y=w224:dbl)
        n182 = Subtract(x=w221, y=w218) -> (x-y=w216:i32)
        n183 = Divide(x=w219, y=w218) -> (x/y=w217:dbl)
        n184 = Multiply(x=w217, y=w216) -> (x*y=w214:dbl)
        "remaining" <- w214
        n185 = Multiply(x=w224, y=100.0) -> (x*y=→"Progress":dbl)
        n186 = Add(x=w215, y=w214) -> (x+y=→"ETA":timestamp)
      }
      frame "end" {
        n187 = Close File(refnum=w464) -> ()  [unwired: 1 in, 2 out]
        n188 = Close File(refnum=w462) -> (path=w461:path)  [unwired: 1 in, 1 out]
        n189 = local write "Status"("finishing" ("Status")) -> ()
        n190 = call "STSGrid.vi"("Binary Spectroscopy File"=w461) -> ()  [unwired: 11 in]
        n191 = Bundle(w469, w469) -> (w491:cluster{sgl[][], sgl[][]})  [unwired: 1 in]
        n192 = Build Array(w491) -> (w490:cluster{sgl[][], sgl[][]}[])
        n193 = Unbundle By Name(w479) -> ("center X (m)"=w477:sgl, "center Y (m)"=w476:sgl, "angle (deg)"=w475:sgl, "width (m)"=w474:sgl, "height (m)"=w473:sgl)
        n194 = Strip Path(path=w449) -> (stripped path=w483:path, name=w482:string)
        n195 = Get Date/Time In Seconds() -> (seconds since 1Jan1904=w445:timestamp)
        n196 = Bundle By Name(cluster=T6 {"up/down"=FALSE, "time/line"=0.0, "start time"=timestamp(0 s since 1904-01-01), "end time"=timestamp(0 s since 1904-01-01)} ("Scan param"), "up/down"=TRUE, "time/line"=sgl nan ("input 7"), "start time"=w487, "end time"=w445) -> (w486:T6)
        n197 = Bundle By Name(cluster=T4 {"center X"=0.0, "center Y"=0.0, "angle"=0.0, "width"=0.0, "height"=0.0, "# pixels"=0, "# lines"=0} ("Scanfield"), "center X"=w477, "center Y"=w476, "angle"=w475, "width"=w474, "height"=w473, "# lines"=w470, "# pixels"=w471) -> (w472:T4)
        n198 = Bundle("stripped path"=w483, "name"=w482) -> (w481:cluster{"stripped path":path, "name":string})  [unwired: 1 in]
        n199 = call <userlib>:"Save sxm File.vi"("Auto file naming? (T)"=FALSE, "Scanfield"=w472, "Scan param"=w486, "error in (no error)"=w480, "Channels data"=w490, "Channels config"=T5 [{"Name"="Z (m)", "Calibration"=1.0, "Offset"=0.0, "Channel index"=0}], "Filename control"=w481) -> ("error out"=w456:errorcluster)  [unwired: 2 in, 2 out]
        n200 = Strip Path(path=w449) -> (stripped path=w460:path)  [unwired: 1 out]
        n201 = Strip Path(path=w460) -> (stripped path=w459:path)  [unwired: 1 out]
        n202 = call <userlib>:"Get Session Path.vi"("error in (no error)"=w456, "Application ref in"=w455) -> ("error out"=w452:errorcluster, "Session path"=w454:path, "Application ref out"=w438:refnum<vi>)  [unwired: 7 in]
        n203 = Path To String(path=w449) -> (string=w448:string)
        n204 = Path To String(path=w459) -> (string=w457:string)
        n205 = call "SXM.vi"("Path"=w454, "Delete"=FALSE, "error in"=w452) -> ("error out"=w451:errorcluster)  [unwired: 7 in]
        n206 = call "ChangeSessionV2.vi"("error in (no error)"=w451, "Session"=w457) -> ("error out"=w450:errorcluster)
        n207 = Format Date/Time String(time format string (%c)=" Finished at %y%m%d - %H%M%S ", seconds (now)=w445) -> (date/time string=w444:string)  [unwired: 1 in]
        n208 = Concatenate Strings(w448, "\r\n", w444) -> (w447:string)
        n209 = Search and Replace String(input string="Email when finished", search string="@") -> (number of replacements=w440:i32)  [unwired: 6 in, 3 out]
        n210 = Greater Than 0?(x=w440) -> (x > 0?=w439:bool)
        n211 = case shown="True" w439 {
          tunnel: w450 -> [_ w498]
          tunnel: w447 -> [_ w496]
          tunnel: "Email when finished" -> [_ w495]
          frame False {
          }
          frame True {
            n212 = call "Send Email"("error in"=w498, "Message"=w496, "Subject"="Grid Finished", "Recipients"=w495) -> ()  [unwired: 7 in, 1 out]
          }
        }
        n213 = local read "Imaging Bias"() -> (w427:dbl)
        n214 = call <userlib>:"BiasSpectroscopy SetProperties.vi"("Application ref in"=w438, "Z-Controller hold (no change)"=enum16{"no change", "on", "off"}."on") -> ("Application ref out"=w436:refnum<vi>)  [unwired: 12 in, 1 out]
        n215 = call <userlib>:"TipLift Set.vi"("TipLift (m)"=sgl 0.0, "Application ref in"=w436) -> ("Application ref out"=w432:refnum<vi>)  [unwired: 8 in, 1 out]
        n216 = call "move2mark (SubVI).vi"("Application in"=w432) -> ("Application out"=w428:refnum<vi>)  [unwired: 10 in]
        n217 = call <userlib>:"Voltage Set.vi"("Bias (V)"=w427, "Application ref in"=w428) -> ("Application ref out"=w429:refnum<vi>)  [unwired: 8 in, 1 out]
        n218 = call <userlib>:"Ctrl-on_off Set.vi"("Z Controller ON/OFF"=TRUE, "Application ref in"=w429) -> ("Application ref out"=w431:refnum<vi>)  [unwired: 8 in, 1 out]
        n219 = call <userlib>:"Point Erase.vi"("Application ref in"=w431, "Point index (-1=All points)"=-1) -> ("Application ref out"=w433:refnum<vi>)  [unwired: 12 in, 1 out]
      }
    }
    "Error out" <- w42
    "Points taken" <- w10
    "X Offset" <- w9
    "Y Offset" <- w8
  }
